vi "Get Suggested Troubleshooting.vi"(8 "error in (no error)":errorcluster, 11 "Current State":T1) -> (0 "error out":errorcluster, 2 "Test Error":errorcluster, 3 "Suggested Troubleshooting":string)   [LabVIEW 2014]
uses:
  Controls/States.ctl
  Globals/Suggested Troubleshooting from R&D.vi
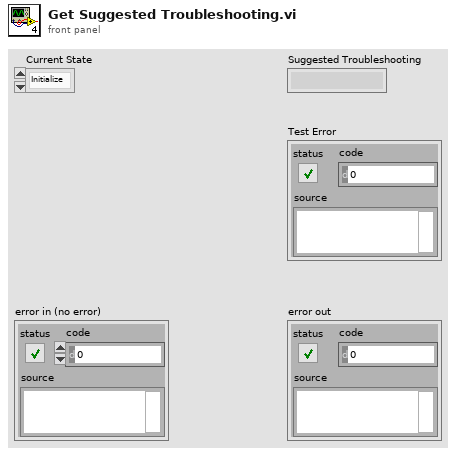
[diagram p1: front panel]
types:
  T1 = typedef "States.ctl" = enum16{"Initialize", "Wait for User Input", "Check User Input", "Insert Open VI", "Run Open VI", "Straight Line", "Home", "Limit", "Generate Report", "Finalize", "Terminate"}
  T2 = cluster{"Test Type":T1, "Troubleshooting List":cluster{"Error Number":i32, "Suggested Troubleshooting":string}[]}[]
  T3 = cluster{"Error Number":i32, "Suggested Troubleshooting":string}[]
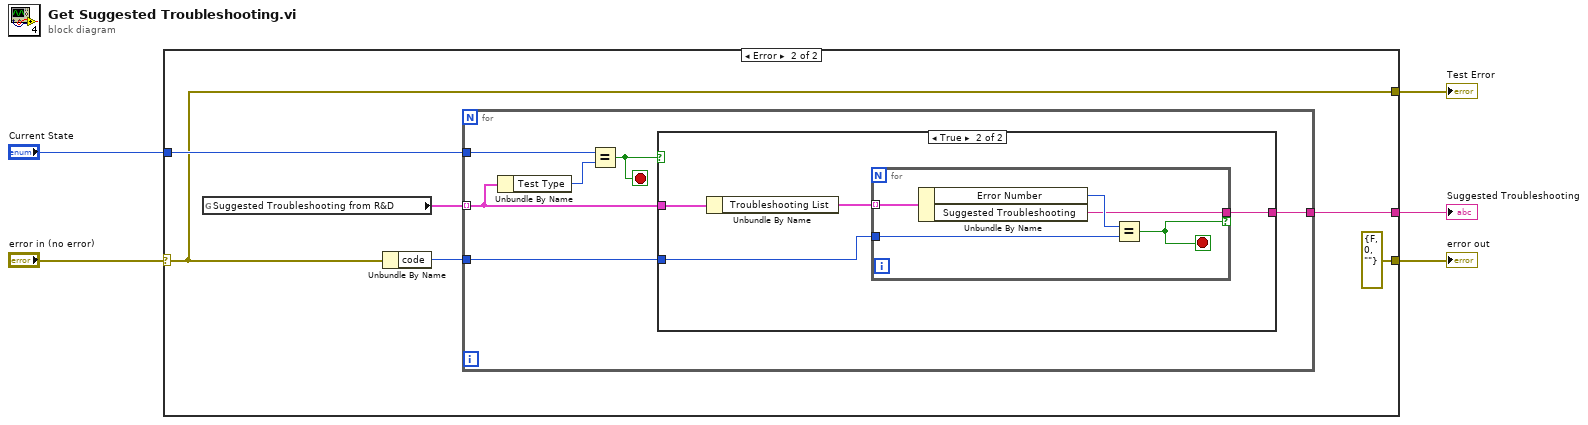
[diagram p0: block diagram]
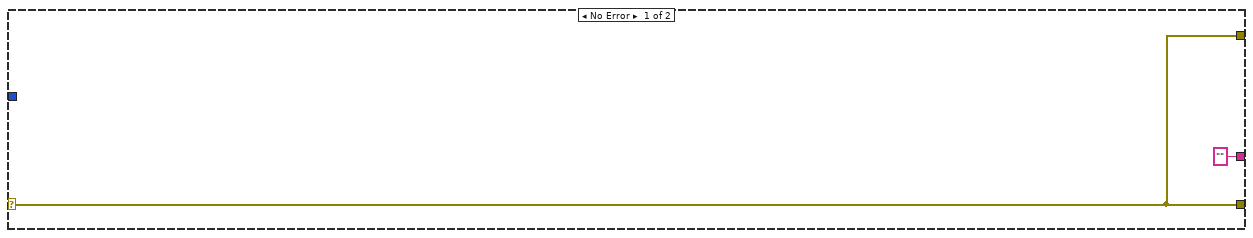
[diagram p2: hidden frame]
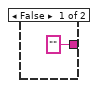
[diagram p3: hidden frame]
diagram:
  n1 = case shown="Error" "error in (no error)" {
    selector: "error in (no error)" -> [w6 w8]
    tunnel: ["" ("Suggested Troubleshooting") w13] -> w2
    tunnel: "Current State" -> [_ w12]
    tunnel: [w6 errorcluster {"status"=FALSE, "code"=0, "source"=""} ("error IO")] -> w4
    tunnel: [w6 w8] -> w1
    frame No Error {
    }
    frame Error {
      n2 = global read "Suggested Troubleshooting from R&D.vi" "Suggested Troubleshooting from R&D"() -> (w11:T2)
      n3 = Unbundle By Name(w8) -> ("code"=w10:i32)
      n4 = for {
        tunnel: w11 -> [w18] mode=indexing
        tunnel: w10 -> [w19]
        tunnel: [w17] -> w13
        tunnel: w12 -> [w15]
        stop <- w14 stop-if-true
        n5 = Unbundle By Name(w18) -> ("Test Type"=w16:T1)
        n6 = Equal?(x=w15, y=w16) -> (x = y?=w14:bool)
        n7 = case shown="True" w14 {
          tunnel: w19 -> [_ w24]
          tunnel: w18 -> [_ w23]
          tunnel: ["" ("Suggested Troubleshooting") w21] -> w17
          frame False {
          }
          frame True {
            n8 = Unbundle By Name(w23) -> ("Troubleshooting List"=w22:T3)
            n9 = for {
              tunnel: w24 -> [w29]
              tunnel: w22 -> [w28] mode=indexing
              tunnel: [w26] -> w21 if=w25
              stop <- w25 stop-if-true
              n10 = Unbundle By Name(w28) -> ("Error Number"=w27:i32, "Suggested Troubleshooting"=w26:string)
              n11 = Equal?(x=w27, y=w29) -> (x = y?=w25:bool)
            }
          }
        }
      }
    }
  }
  "error out" <- w4
  "Suggested Troubleshooting" <- w2
  "Test Error" <- w1
